vi "S3Outputs.vi"(8 "error in":errorcluster, 11 "SIOutputs":T1={"LO P"=FALSE, "HI P"=FALSE, "Z3Vent"=FALSE, "V2 Vent"=FALSE, "IsLidLocked"=TRUE}) -> (0 "error out":errorcluster)   [LabVIEW 2018, in "IO.lvclass"]
uses:
  IO.lvclass
  S3/Public Controls/Outputs.ctl
  Queue/Queue Data.ctl
  Queue/State.ctl
  3f94d1a5-99fd-4959-a653-d214a615357f.vi
  S3/S3.lvclass
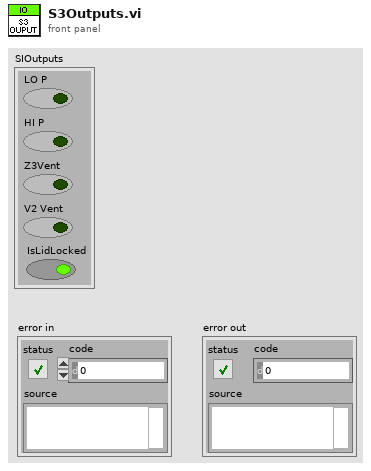
[diagram p1: front panel]
types:
  T1 = typedef "S3.lvclass/Outputs.ctl" = cluster{"LO P":bool, "HI P":bool, "Z3Vent":bool, "V2 Vent":bool, "IsLidLocked":bool}
  T2 = typedef "IO.lvclass/Queue Data.ctl" = cluster{"State":T3, "Data":variant}
  T3 = typedef "IO.lvclass/State.ctl" = enum16{"Initialize", "GlobalConfig", "ESTOP", "Abort", "S1Ouputs", "S2Outputs", "S3Ouputs", "S4Outputs", "S5Outputs", "S6Outputs", "Read", "Error", "Exit"}
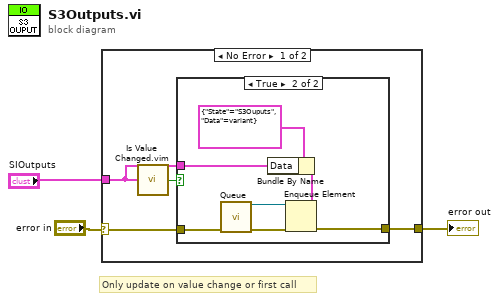
[diagram p0: block diagram]
diagram:
  # "Only update on value change or first call"
  n1 = case shown="No Error" "error in" {
    selector: "error in" -> [w7 w16]
    tunnel: [w6 w16] -> w3
    tunnel: "SIOutputs" -> [w4 _]
    frame No Error {
      n2 = call "Is Value Changed.vim"("value"=w4) -> ("changed or first call?"=w5:bool)
      n3 = case shown="True" w5 {
        tunnel: w7 -> [w8 w15]
        tunnel: [w8 w12] -> w6
        tunnel: w4 -> [_ w9]
        frame False {
        }
        frame True {
          n4 = call "Queue.vi"("error in"=w15) -> ("error out"=w14:errorcluster, "queue out"=w13:refnum<queue>)  [unwired: 9 in]
          n5 = Bundle By Name(cluster=T2 {"State"=enum."S3Ouputs", "Data"=variant} ("element"), "Data"=w9) -> (w10:T2)
          n6 = Enqueue Element(queue=w13, element=w10, error in (no error)=w14) -> (error out=w12:errorcluster)  [unwired: 1 in, 2 out]
        }
      }
    }
    frame Error {
    }
  }
  "error out" <- w3
